vi "XML to Physical Constants.vi"(0 "XML Data":string) -> ()   [LabVIEW 2013]
uses:
  Types/Physical Constants.ctl
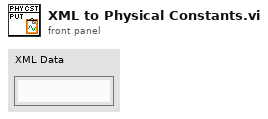
[diagram p1: front panel]
types:
  T1 = typedef "Physical Constants.ctl" = cluster{"Maximum Input Voltage":dbl, "Maximum Output Voltage":dbl, "Minimum Input Voltage":dbl, "Minimum Output Voltage":dbl, "X Maximum Extension":dbl, "X Minimum Extension":dbl, "X Piezo Response":dbl, "Y Maximum Extension":dbl, "Y Minimum Extension":dbl, "Y Piezo Response":dbl, "Z Maximum Extension":dbl, "Z Minimum Extension":dbl, "Z Piezo Response":dbl, "Version":string}
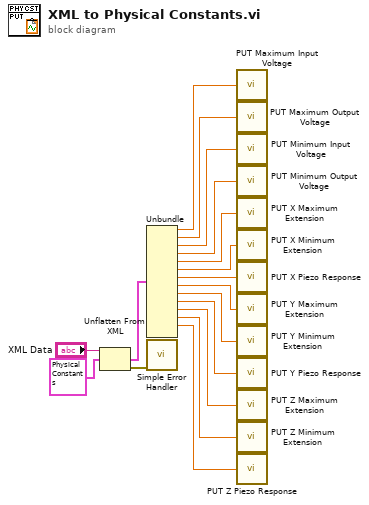
[diagram p0: block diagram]
diagram:
  n1 = Unflatten From XML(xml string="XML Data", type=T1 {"Maximum Input Voltage"=0.0, "Maximum Output Voltage"=0.0, "Minimum Input Voltage"=0.0, "Minimum Output Voltage"=0.0, "X Maximum Extension"=0.0, "X Minimum Extension"=0.0, "X Piezo Response"=0.0, "Y Maximum Extension"=0.0, "Y Minimum Extension"=0.0, "Y Piezo Response"=0.0, "Z Maximum Extension"=0.0, "Z Minimum Extension"=0.0, "Z Piezo Response"=0.0, "Version"=""} ("Physical Constants")) -> (value=w14:T1, error out=w17:errorcluster)  [unwired: 1 in]
  n2 = Unbundle(w14) -> ("Maximum Input Voltage"=w7:dbl, "Maximum Output Voltage"=w8:dbl, "Minimum Input Voltage"=w9:dbl, "Minimum Output Voltage"=w10:dbl, "X Maximum Extension"=w11:dbl, "X Minimum Extension"=w12:dbl, "X Piezo Response"=w13:dbl, "Y Maximum Extension"=w6:dbl, "Y Minimum Extension"=w5:dbl, "Y Piezo Response"=w4:dbl, "Z Maximum Extension"=w3:dbl, "Z Minimum Extension"=w2:dbl, "Z Piezo Response"=w1:dbl)  [unwired: 1 out]
  n3 = call <vilib>:"Simple Error Handler.vi"("error in (no error)"=w17) -> ()  [unwired: 4 in, 5 out]
  n4 = call "PUT Maximum Input Voltage.vi"("Maximum Input Voltage"=w7) -> ()
  n5 = call "PUT Maximum Output Voltage.vi"("Maximum Output Voltage"=w8) -> ()
  n6 = call "PUT Minimum Input Voltage.vi"("Minimum Input Voltage"=w9) -> ()
  n7 = call "PUT Minimum Output Voltage.vi"("Minimum Output Voltage"=w10) -> ()
  n8 = call "PUT X Maximum Extension.vi"("X Maximum Extension"=w11) -> ()
  n9 = call "PUT X Minimum Extension.vi"("X Minimum Extension"=w12) -> ()
  n10 = call "PUT X Piezo Response.vi"("X Piezo Response"=w13) -> ()
  n11 = call "PUT Y Maximum Extension.vi"("Y Maximum Extension"=w6) -> ()
  n12 = call "PUT Y Minimum Extension.vi"("Y Minimum Extension"=w5) -> ()
  n13 = call "PUT Y Piezo Response.vi"("Y Piezo Response"=w4) -> ()
  n14 = call "PUT Z Maximum Extension.vi"("Z Maximum Extension"=w3) -> ()
  n15 = call "PUT Z Minimum Extension.vi"("Z Minimum Extension"=w2) -> ()
  n16 = call "PUT Z Piezo Response.vi"("Z Piezo Response"=w1) -> ()
